vi "F Dwf Analog Out Phase Info.vi"(7 "pdegreeMax":dbl, 8 "error in (no error)":errorcluster, 9 "pdegreeMin":dbl, 10 "idxChannel":i32, 11 "hdwf":i32) -> (0 "error out":errorcluster, 1 "pdegreeMin out":dbl, 3 "function return":i32, 5 "pdegreeMax out":dbl)   [LabVIEW 2019, in "Olasdwf.lvlib"]
doc: "DWFAPI int FDwfAnalogOutPhaseInfo(HDWF hdwf, int idxChannel, double *pdegreeMin, double *pdegreeMax);"
uses:
  Olasdwf.lvlib
  Windows/System32/dwf.dll
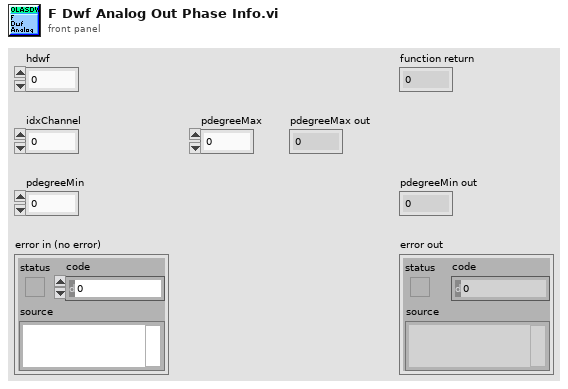
[diagram p1: front panel]
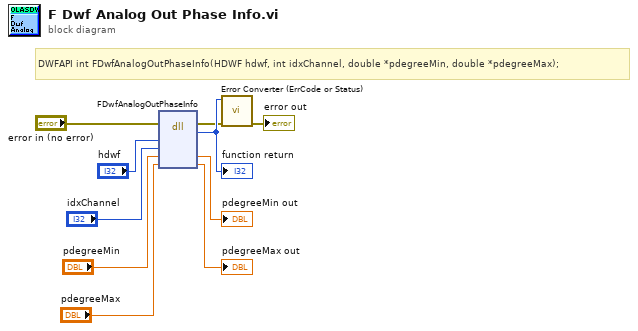
[diagram p0: block diagram]
diagram:
  # "DWFAPI int FDwfAnalogOutPhaseInfo(HDWF hdwf, int idxChannel, double *pdegreeMin, double *pdegreeMax);"
  n1 = dll-call lib="C:/Windows/System32/dwf.*" fn="FDwfAnalogOutPhaseInfo"(error in="error in (no error)", "hdwf"="hdwf", "idxChannel"="idxChannel", "pdegreeMin"="pdegreeMin", "pdegreeMax"="pdegreeMax") -> (error out=w2:errorcluster, w10:i32, "pdegreeMin"=→"pdegreeMin out":dbl, "pdegreeMax"=→"pdegreeMax out":dbl)  [unwired: 4 in, 1 out]
  "function return" <- w10
  n2 = call "Error Converter (ErrCode or Status).vi"("error in (no error)"=w2, "error code"=w10) -> ("error out"=→"error out":errorcluster)  [unwired: 9 in]
